vi "rdb_json_elements_to_cluster.vi"(8 "error in (no error)":errorcluster, 9 "index (0)":i32, 10 "indent (0)":i32, 11 "elements":T1[](array[typedef])) -> (0 "error out":errorcluster, 1 "index out":i32, 3 "variant":variant)   [LabVIEW 2017]
uses:
  rdb_json_element.ctl
  rdb_json_type.ctl
panel:
  in  "containers":cluster{"key":string, "elements":variant[]}[](array[cluster])
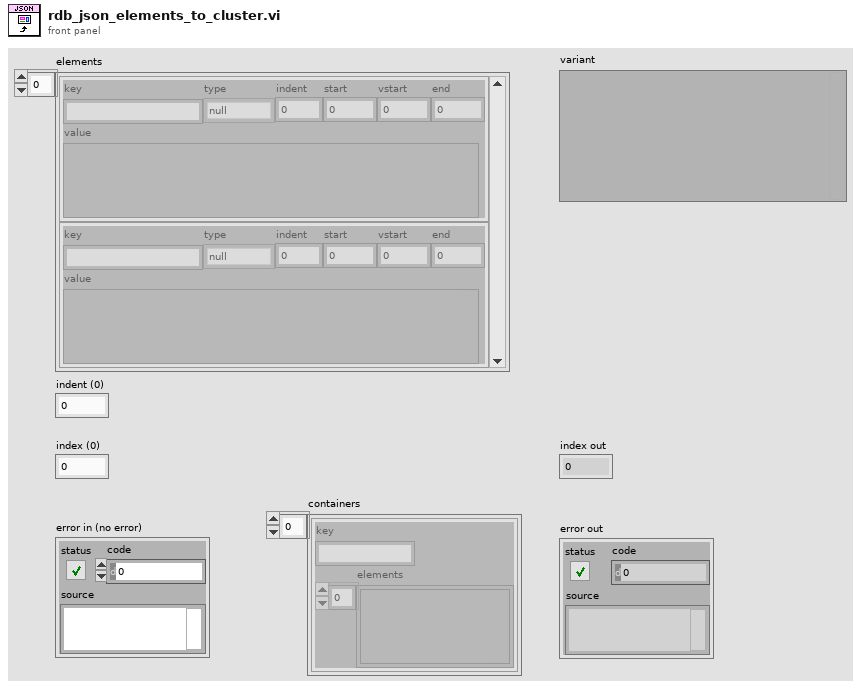
[diagram p1: front panel]
types:
  T1 = typedef "rdb_json_element.ctl" = cluster{"key":string, "type":T2, "indent":i32, "start":i32, "vstart":i32, "end":i32, "value":variant}
  T2 = typedef "rdb_json_type.ctl" = enum8{"null", "bool", "int", "uint", "float", "string", "array", "object", "invalid"}
  T3 = cluster{"t":enum8{"object", "array"}, "k":string, "e":variant[]}[]
  T4 = cluster{"t":enum8{"object", "array"}, "k":string, "e":variant[]}
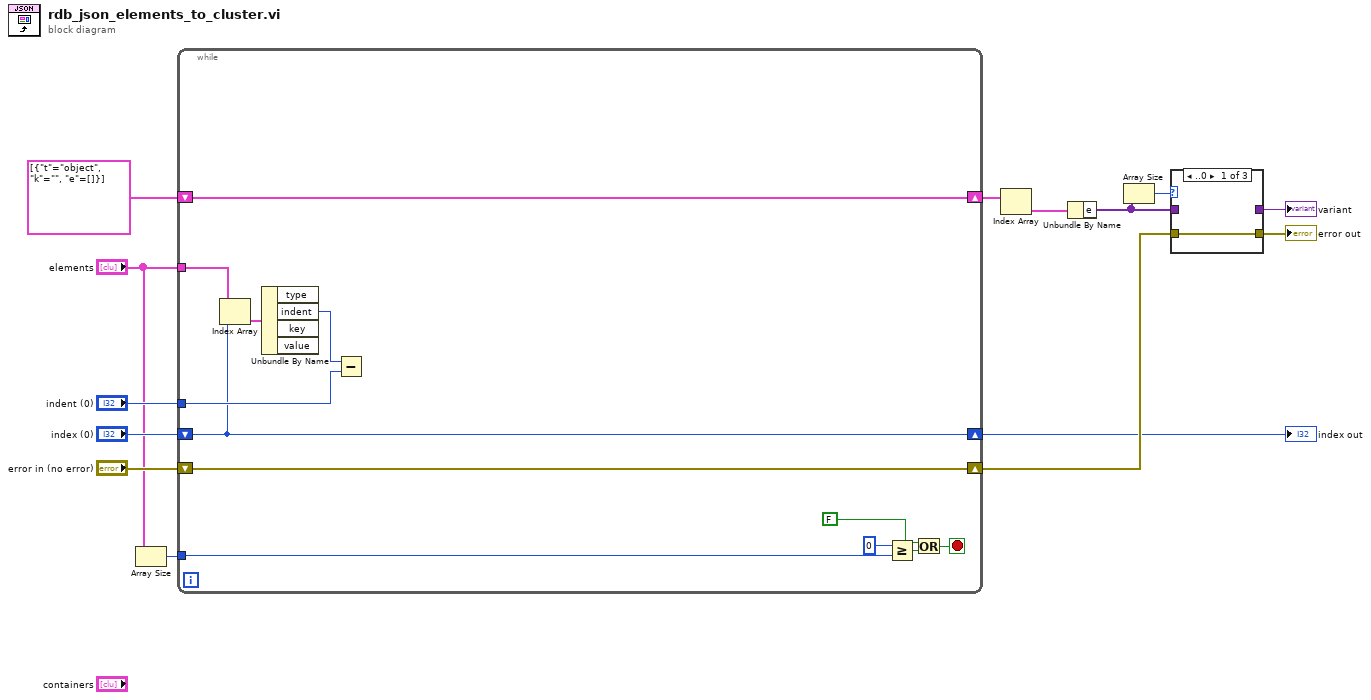
[diagram p0: block diagram]
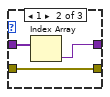
[diagram p2: hidden frame]
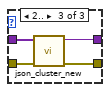
[diagram p3: hidden frame]
diagram:
  n1 = Array Size(array="elements") -> (size(s)=w6:i32)
  n2 = while {
    tunnel: "elements" -> [w26]
    shift-right: [w17] -> w11
    shift-left: "error in (no error)" -> [w17]
    tunnel: "indent (0)" -> [w20]
    tunnel: w6 -> [w25]
    shift-right: [w18] -> w5
    shift-left: "index (0)" -> [w18]
    shift-right: [w19] -> w3
    shift-left: T3 [{"t"=enum."object", "k"="", "e"=[]}] ("indents") -> [w19]
    stop <- w24 stop-if-true
    n3 = Index Array(array=w26, index=w18) -> (element=w23:T1)
    n4 = Unbundle By Name(w23) -> ("indent"=w21:i32)  [unwired: 3 out]
    n5 = Subtract(x=w21, y=w20) -> ()  [unwired: 1 out]
    n6 = Greater Or Equal?(x=0, y=w25) -> (x >= y?=w22:bool)
    n7 = Or(x=FALSE, y=w22) -> (x .or. y?=w24:bool)
  }
  "index out" <- w5
  n8 = Index Array(array=w3) -> (element=w2:T4)  [unwired: 1 in]
  n9 = Unbundle By Name(w2) -> ("e"=w1:variant[])
  n10 = Array Size(array=w1) -> (size(s)=w9:i32)
  n11 = case shown="..0" w9 {
    tunnel: w1 -> [_ w30 w34]
    tunnel: w11 -> [w27 w28 w33]
    tunnel: [w27 w28 w32] -> w10
    tunnel: [_ w29 w31] -> w8
    frame ..0 {
    }
    frame 1 {
      n12 = Index Array(array=w30) -> (element=w29:variant)  [unwired: 1 in]
    }
    frame 2.. {
      n13 = call "json_cluster_new.vi"("error in (no error)"=w33, "elements"=w34) -> ("error out"=w32:errorcluster, "cluster"=w31:variant)  [unwired: 8 in]
    }
  }
  "error out" <- w10
  "variant" <- w8
